vi "Get Routine Object.vi"(7 "Settings":T2=enum."Custom", 8 "error in (no error)":errorcluster, 10 "6 Inch":bool, 11 "Routine":T1=enum."Secure Syringe") -> (0 "error out":errorcluster, 3 "Routine out":refnum<class "Routine.lvclass">)   [LabVIEW 2019, in "Routine.lvclass"]
uses:
  Routine.lvclass
  Settings.ctl
  Routine Enum.ctl
  Dispense/Iterative Dispense/Glue Step Enum.ctl
  Dispense/Iterative Dispense/8 inch/8 Inch Iterative Dispense.lvclass
  C:/Users/HEP/Documents/Aerotech gantry/UCSB-Gantry-master-main/V5/Classes/Routine/Dispense/Iterative Dispense/Iterative Dispense.lvclass
  Dispense/Iterative Dispense/6 inch/6 Inch Iterative Dispense.lvclass
  Dispense/Iterative Dispense/Iterative Dispense.lvclass/Iterative Dispense.ctl
  Dispense/CAD Dispense/8 Inch CAD Dispense.lvclass
  C:/Users/HEP/Documents/Aerotech gantry/UCSB-Gantry-master-main/V5/Classes/Routine/Dispense/CAD Dispense/CAD Dispense.lvclass
  Dispense/CAD Dispense/6 inch CAD Dispense.lvclass
  Dispense/CAD Dispense/Offset Dispense.lvclass
  C:/Users/HEP/Documents/Aerotech gantry/UCSB-Gantry-master-main/V5/Classes/Routine/Routine.lvclass
  Pick and Place/Pick and Place.lvclass
  Pick and Place/Pick and Place Type.ctl
  Pick and Place/Pick and Place.lvclass/Pick and Place.ctl
  Secure Syringe/SecureRelease Syringe.lvclass
  Secure Syringe/SecureRelease Syringe.lvclass/SecureRelease Syringe.ctl
  Dispense/Iterative Dispense/Write Glue Step Enum.vi
  Pick and Place/Write Pick and Place Type.vi
  Secure Syringe/Write Type.vi
  Dispense/Iterative Dispense/Iterative Dispense.lvclass
  Dispense/CAD Dispense/CAD Dispense.lvclass
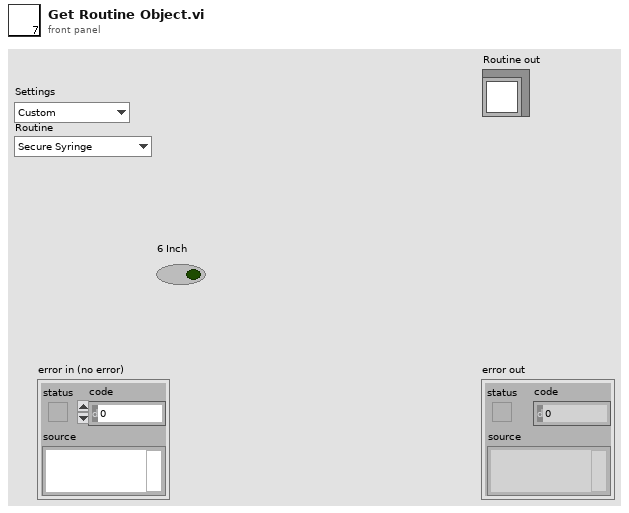
[diagram p1: front panel]
types:
  T1 = typedef "Routine.lvclass/Routine Enum.ctl" = enum16{"Primary Pick Up", "Pick Up All", "Put Down Secondary", "Put Down All", "Release Syringe", "Secondary Pick Up", "Secure Syringe", "Dispense on Plate", "Dispense on Kapton", "Dispense on Sensor", "Dispense Offset"}
  T2 = typedef "Routine.lvclass/Settings.ctl" = enum16{"Default", "Custom"}
  T3 = typedef "Pick and Place.lvclass/Pick and Place Type.ctl" = enum16{"Primary Pick Up", "Secondary Pick Up", "Put Down All", "Pick Up All", "Put Down Secondary"}
  T4 = typedef "Iterative Dispense.lvclass/Glue Step Enum.ctl" = enum16{"Baseplate to Kapton", "Kapton to Sensor"}
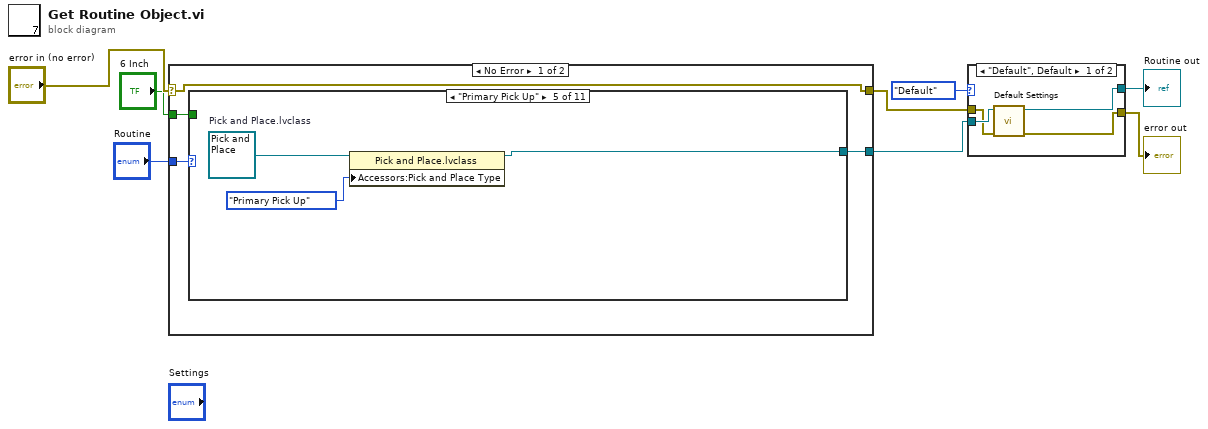
[diagram p0: block diagram]
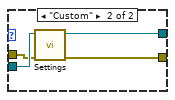
[diagram p2: hidden frame]
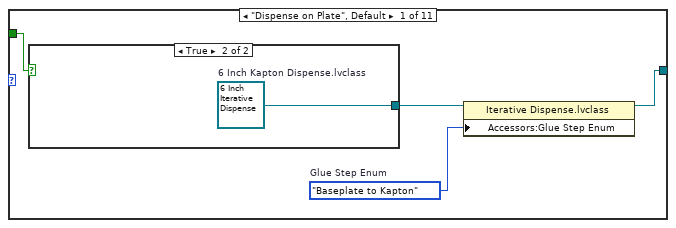
[diagram p3: hidden frame]
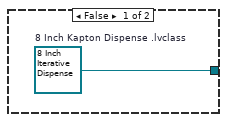
[diagram p4: hidden frame]
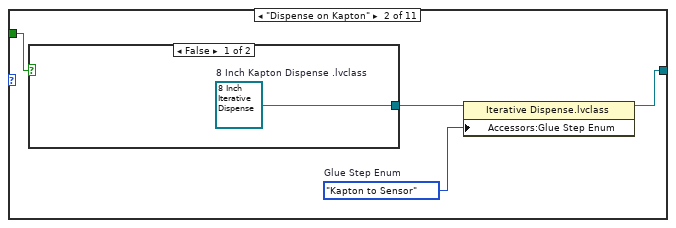
[diagram p5: hidden frame]
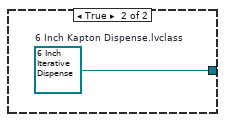
[diagram p6: hidden frame]
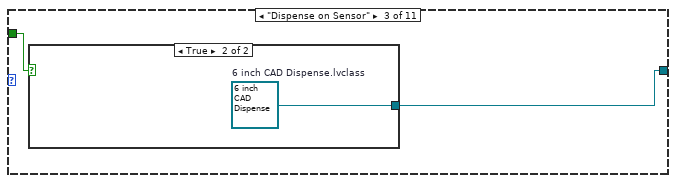
[diagram p7: hidden frame]
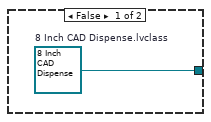
[diagram p8: hidden frame]
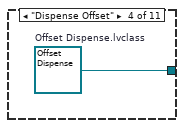
[diagram p9: hidden frame]
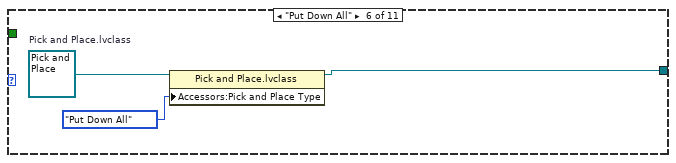
[diagram p10: hidden frame]
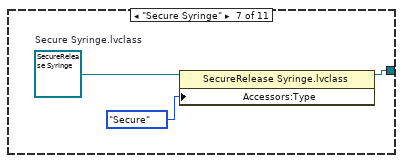
[diagram p11: hidden frame]
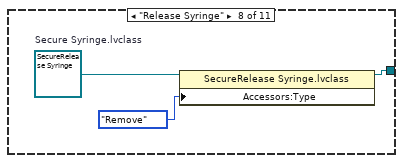
[diagram p12: hidden frame]
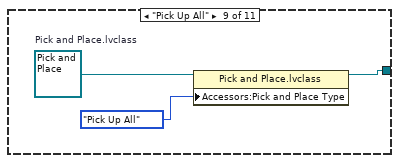
[diagram p13: hidden frame]
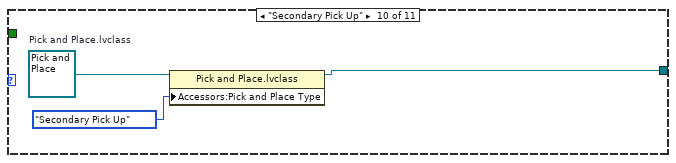
[diagram p14: hidden frame]
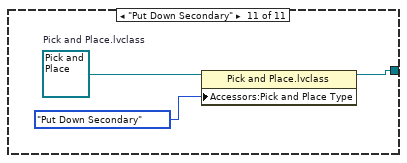
[diagram p15: hidden frame]
diagram:
  n1 = case shown="No Error" "error in (no error)" {
    selector: "error in (no error)" -> [w12 w51]
    tunnel: [w12 w51] -> w2
    tunnel: [w11 _] -> w7
    tunnel: "Routine" -> [w10 _]
    tunnel: "6 Inch" -> [w9 _]
    frame No Error {
      n2 = case shown="\"Primary Pick Up\"" w10 {
        tunnel: [w16 w22 w26 w29 w31 w34 w36 w39 w42 w45 w48] -> w11
        tunnel: w9 -> [w14 w20 w25 _ _ _ _ _ _ _ _]
        frame "Dispense on Plate", Default {
          w15 = Glue_Step_Enum."Baseplate to Kapton"  # Glue Step Enum
          n3 = case shown="True" w14 {
            tunnel: [w17 w18] -> w13
            frame False {
              w17 = refnum<class "8 Inch Iterative Dispense.lvclass"> refnum  # 8 Inch Kapton Dispense .lvclass
            }
            frame True {
              w18 = refnum<class "6 Inch Iterative Dispense.lvclass"> refnum  # 6 Inch Kapton Dispense.lvclass
            }
          }
          n4 = property class="Iterative Dispense.lvclass"(reference=w13, "Accessors:Glue Step Enum"=w15) -> (reference out=w16:refnum<class "Iterative Dispense.lvclass">)  [unwired: 1 in, 1 out]
        }
        frame "Dispense on Kapton" {
          w21 = Glue_Step_Enum."Kapton to Sensor"  # Glue Step Enum
          n5 = case shown="False" w20 {
            tunnel: [w23 w24] -> w19
            frame False {
              w23 = refnum<class "8 Inch Iterative Dispense.lvclass"> refnum  # 8 Inch Kapton Dispense .lvclass
            }
            frame True {
              w24 = refnum<class "6 Inch Iterative Dispense.lvclass"> refnum  # 6 Inch Kapton Dispense.lvclass
            }
          }
          n6 = property class="Iterative Dispense.lvclass"(reference=w19, "Accessors:Glue Step Enum"=w21) -> (reference out=w22:refnum<class "Iterative Dispense.lvclass">)  [unwired: 1 in, 1 out]
        }
        frame "Dispense on Sensor" {
          n7 = case shown="True" w25 {
            tunnel: [w27 w28] -> w26
            frame False {
              w27 = refnum<class "8 Inch CAD Dispense.lvclass"> refnum  # 8 Inch CAD Dispense.lvclass
            }
            frame True {
              w28 = refnum<class "6 inch CAD Dispense.lvclass"> refnum  # 6 inch CAD Dispense.lvclass
            }
          }
        }
        frame "Dispense Offset" {
          w29 = refnum<class "Offset Dispense.lvclass"> refnum  # Offset Dispense.lvclass
        }
        frame "Primary Pick Up" {
          w32 = refnum<class "Pick and Place.lvclass"> refnum  # Pick and Place.lvclass
          n8 = property class="Pick and Place.lvclass"(reference=w32, "Accessors:Pick and Place Type"=Pick_and_Place_Type."Primary Pick Up" ("Pick and Place Type")) -> (reference out=w31:refnum<class "Pick and Place.lvclass">)  [unwired: 1 in, 1 out]
        }
        frame "Put Down All" {
          w35 = refnum<class "Pick and Place.lvclass"> refnum  # Pick and Place.lvclass
          n9 = property class="Pick and Place.lvclass"(reference=w35, "Accessors:Pick and Place Type"=Pick_and_Place_Type."Put Down All" ("Pick and Place Type")) -> (reference out=w34:refnum<class "Pick and Place.lvclass">)  [unwired: 1 in, 1 out]
        }
        frame "Secure Syringe" {
          w38 = refnum<class "SecureRelease Syringe.lvclass"> refnum  # Secure Syringe.lvclass
          n10 = property class="SecureRelease Syringe.lvclass"(reference=w38, "Accessors:Type"=enum16{"Secure", "Remove"}."Secure" ("Type")) -> (reference out=w36:refnum<class "SecureRelease Syringe.lvclass">)  [unwired: 1 in, 1 out]
        }
        frame "Release Syringe" {
          w41 = refnum<class "SecureRelease Syringe.lvclass"> refnum  # Secure Syringe.lvclass
          n11 = property class="SecureRelease Syringe.lvclass"(reference=w41, "Accessors:Type"=enum16{"Secure", "Remove"}."Remove" ("Type")) -> (reference out=w39:refnum<class "SecureRelease Syringe.lvclass">)  [unwired: 1 in, 1 out]
        }
        frame "Pick Up All" {
          w44 = refnum<class "Pick and Place.lvclass"> refnum  # Pick and Place.lvclass
          n12 = property class="Pick and Place.lvclass"(reference=w44, "Accessors:Pick and Place Type"=Pick_and_Place_Type."Pick Up All" ("Pick and Place Type")) -> (reference out=w42:refnum<class "Pick and Place.lvclass">)  [unwired: 1 in, 1 out]
        }
        frame "Secondary Pick Up" {
          w47 = refnum<class "Pick and Place.lvclass"> refnum  # Pick and Place.lvclass
          n13 = property class="Pick and Place.lvclass"(reference=w47, "Accessors:Pick and Place Type"=Pick_and_Place_Type."Secondary Pick Up" ("Pick and Place Type")) -> (reference out=w45:refnum<class "Pick and Place.lvclass">)  [unwired: 1 in, 1 out]
        }
        frame "Put Down Secondary" {
          w50 = refnum<class "Pick and Place.lvclass"> refnum  # Pick and Place.lvclass
          n14 = property class="Pick and Place.lvclass"(reference=w50, "Accessors:Pick and Place Type"=Pick_and_Place_Type."Put Down Secondary" ("Pick and Place Type")) -> (reference out=w48:refnum<class "Pick and Place.lvclass">)  [unwired: 1 in, 1 out]
        }
      }
    }
    frame Error {
    }
  }
  n15 = case shown="\"Default\", Default" Settings."Default" ("Settings") {
    tunnel: w7 -> [w55 w59]
    tunnel: [w54 w58] -> w6
    tunnel: w2 -> [w53 w57]
    tunnel: [w52 w56] -> w1
    frame "Default", Default {
      n16 = call-dynamic "Default Settings.vi"("error in (no error)"=w53, "Routine in"=w55) -> ("error out"=w52:errorcluster, "Routine out"=w54:refnum<class "Routine.lvclass">)  [unwired: 8 in]
    }
    frame "Custom" {
      n17 = call-dynamic "Settings.vi"("error in (no error)"=w57, "Routine in"=w59) -> ("error out"=w56:errorcluster, "Routine out"=w58:refnum<class "Routine.lvclass">)  [unwired: 8 in]
    }
  }
  "error out" <- w1
  "Routine out" <- w6
